vi "Spectrometer Digikröm Control Panel (No Objects).vi"(8 "error in (no error)":errorcluster) -> (0 "error out":errorcluster)   [LabVIEW 2012]
uses:
  <vilib>/Utility/error.llb/DialogType.ctl
  Digikrom DK24x/Digikrom DK24x.lvlib
panel:
  in  "exit":bool
  in  "Control":T1={"Goto Wavelength"=0.0, "Slit 1 width"=1.0000000000000004e-05, "Slit 2 width"=1.0000000000000004e-05, "Filter"=3, "Grating"=1} {"Grating" items=["Grating A"=1, "Grating B"=2, "Grating C"=3]; "Filter" items=["No filter", "Filter 1", "Filter 2", "Filter 3", "Filter 4", "Filter 5"]; "Slit 2 width" min=1.0000000000000004e-05 max=0.005000000000000002 step=1.0000000000000004e-05; "Slit 1 width" min=1.0000000000000004e-05 max=0.005000000000000002 step=1.0000000000000004e-05; "Goto Wavelength" min=0.0 max=6e-06 step=1.0000000000000008e-13 format="%.2f"}
  out "Status":T2={"Ready"=FALSE, "Wavelength"=5.000000000000003e-07, "Entrance slit"=9.999999999999999e-06, "Exit slit"=9.999999999999999e-06, " Grating (nm)"=500.0, " Filter"=0.0} {"Exit slit" format="%.2f"; "Entrance slit" format="%.2f"; "Wavelength" min=0.0 format="%.2f"}
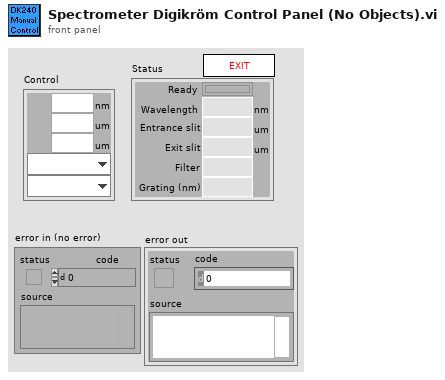
[diagram p1: front panel]
types:
  T1 = cluster{"Goto Wavelength":dbl[unit], "Slit 1 width":dbl[unit], "Slit 2 width":dbl[unit], "Filter":u32, "Grating":u16}
  T2 = cluster{"Ready":bool, "Wavelength":dbl[unit], "Entrance slit":dbl[unit], "Exit slit":dbl[unit], " Grating (nm)":dbl, " Filter":dbl}
  T3 = typedef "DialogType.ctl" = u16
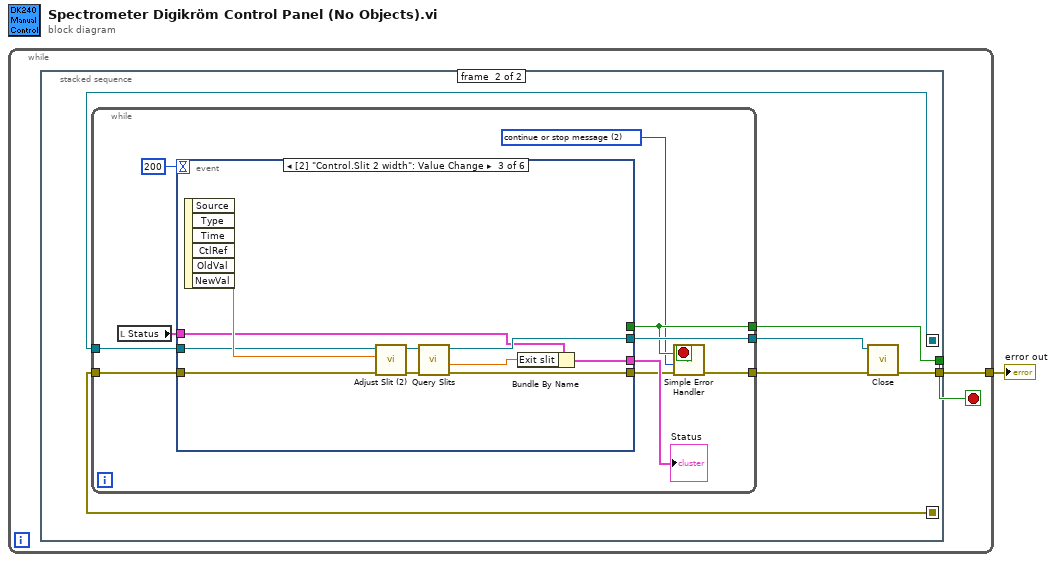
[diagram p0: block diagram]
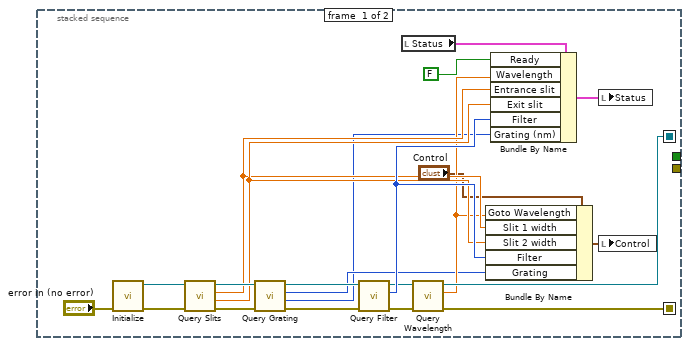
[diagram p2: hidden frame]
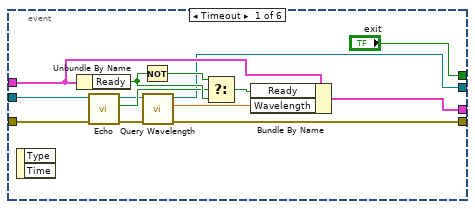
[diagram p3: hidden frame]
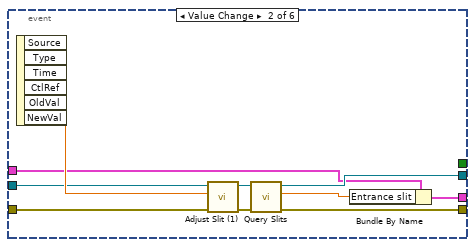
[diagram p4: hidden frame]
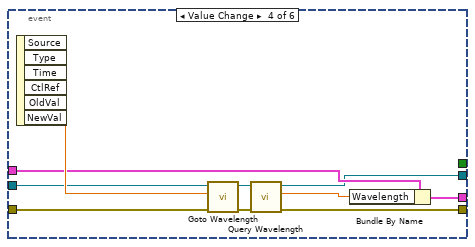
[diagram p5: hidden frame]
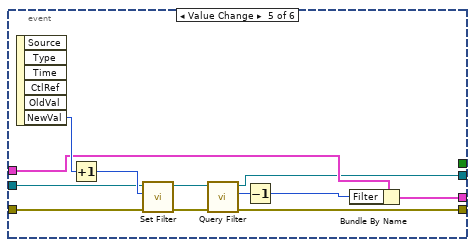
[diagram p6: hidden frame]
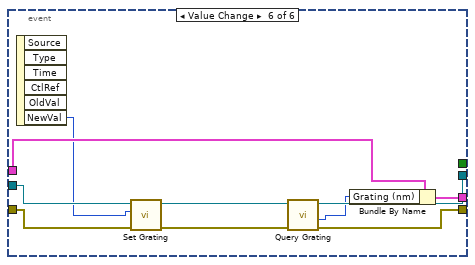
[diagram p7: hidden frame]
diagram:
  n1 = while {
    tunnel: [w2] -> w1
    stop <- w3 stop-if-true
    n2 = stacked-sequence {
      seq-local: [w18 _] -> [_ w30]
      seq-local: [w17 _] -> [_ w31]
      tunnel: [_ w29] -> w3
      tunnel: [_ w26] -> w2
      frame #0 {
        n3 = call "Initialize.vi"("error in (no error)"="error in (no error)") -> ("error out"=w22:errorcluster, "VISA resource name out"=w21:refnum<visa-resource-name>)  [unwired: 2 in, 7 out]
        n4 = call "Query Slits.vi"("error in (no error)"=w22, "VISA resource name"=w21) -> ("error out"=w19:errorcluster, "CURRENT S2 WIDTH"=w14:dbl[unit], "CURRENT S1 WIDTH"=w13:dbl[unit], "VISA resource name out"=w20:refnum<visa-resource-name>)  [unwired: 6 out]
        n5 = call "Query Grating.vi"("error in (no error)"=w19, "VISA resource name"=w20) -> ("error out"=w8:errorcluster, "BLAZE (nm)"=w6:u16, "GRATING #"=w7:u8, "VISA resource name out"=w9:refnum<visa-resource-name>)  [unwired: 6 out]
        n6 = call "Query Filter.vi"("error in (no error)"=w8, "VISA resource name"=w9) -> ("error out"=w10:errorcluster, "CURRENT FILTER"=w15:u8, "VISA resource name out"=w11:refnum<visa-resource-name>)  [unwired: 7 out]
        n7 = local read "Status"() -> (w24:T2)
        n8 = call "Query Wavelength.vi"("error in (no error)"=w10, "VISA resource name"=w11) -> ("error out"=w17:errorcluster, "CURRENT WAVELENGTH"=w12:dbl[unit], "VISA resource name out"=w18:refnum<visa-resource-name>)  [unwired: 7 out]
        n9 = Bundle By Name(cluster="Control", "Goto Wavelength"=w12, "Slit 1 width"=w13, "Slit 2 width"=w14, "Filter"=w15, "Grating"=w7) -> (w23:T1)
        n10 = Bundle By Name(cluster=w24, "Ready"=FALSE, "Wavelength"=w12, "Entrance slit"=w13, "Exit slit"=w14, "Filter"=w15, "Grating (nm)"=w6) -> (w25:T2)
        n11 = local write "Status"(w25) -> ()
        n12 = local write "Control"(w23) -> ()
      }
      frame #1 {
        n13 = while {
          tunnel: [w34] -> w29
          tunnel: w31 -> [w39]
          tunnel: [w33] -> w28
          tunnel: w30 -> [w38]
          tunnel: [w37] -> w27
          stop <- w34 stop-if-true
          w32 = T3 2 items=["no dialog", "OK message", "continue or stop message", "OK message + warnings", "continue/stop + warnings"] ("type of dialog (OK msg:1)")
          n14 = local read "Status"() -> (w35:T2)
          n15 = event shown="[2] \"Control.Slit 2 width\": Value Change" {
            selector: _ -> [_ _ _ _ _ _]
            dyn-events: _ -> [_ _ _ _ _ _]
            timeout: 200 -> [_ _ _ _ _ _]
            tunnel: ["exit" _ _ _ _ _] -> w34
            tunnel: [w55 w65 w75 w84 w96 w107] -> w41
            tunnel: w38 -> [w50 w59 w70 w81 w88 w106]
            tunnel: w39 -> [w51 w60 w71 w82 w92 w105]
            tunnel: [w45 w62 w73 w77 w86 w98] -> w36
            tunnel: [w46 w63 w74 w76 w87 w100] -> w37
            tunnel: w35 -> [w49 w58 w69 w80 w91 w104]
            event Timeout {
              n16 = event-data() -> ()  [unwired: 3 out]
              n17 = Unbundle By Name(w49) -> ("Ready"=w52:bool)
              n18 = call "Echo.vi"("error in (no error)"=w51, "VISA resource name"=w50) -> ("error out"=w44:errorcluster, "Comm OK?"=w48:bool, "VISA resource name out"=w43:refnum<visa-resource-name>)  [unwired: 7 out]
              n19 = Not(x=w52) -> (.not. x?=w53:bool)
              n20 = call "Query Wavelength.vi"("error in (no error)"=w44, "VISA resource name"=w43) -> ("error out"=w45:errorcluster, "CURRENT WAVELENGTH"=w42:dbl[unit], "VISA resource name out"=w46:refnum<visa-resource-name>)  [unwired: 7 out]
              n21 = Select(t=w53, s=w48, f=w52) -> (s? t:f=w54:bool)
              n22 = Bundle By Name(cluster=w49, "Ready"=w54, "Wavelength"=w42) -> (w55:T2)
            }
            event "Control.Slit 1 width": Value Change {
              n23 = event-data() -> ("NewVal"=w61:dbl[unit])  [unwired: 6 out]
              n24 = call "Adjust Slit (1).vi"("error in (no error)"=w60, "SLIT WIDTH"=w61, "VISA resource name"=w59) -> ("error out"=w57:errorcluster, "VISA resource name out"=w56:refnum<visa-resource-name>)  [unwired: 7 out]
              n25 = call "Query Slits.vi"("error in (no error)"=w57, "VISA resource name"=w56) -> ("error out"=w62:errorcluster, "CURRENT S1 WIDTH"=w64:dbl[unit], "VISA resource name out"=w63:refnum<visa-resource-name>)  [unwired: 7 out]
              n26 = Bundle By Name(cluster=w58, "Entrance slit"=w64) -> (w65:T2)
            }
            event "Control.Slit 2 width": Value Change {
              n27 = event-data() -> ("NewVal"=w72:dbl[unit])  [unwired: 6 out]
              n28 = call "Adjust Slit (2).vi"("error in (no error)"=w71, "SLIT WIDTH"=w72, "VISA resource name"=w70) -> ("error out"=w68:errorcluster, "VISA resource name out"=w67:refnum<visa-resource-name>)  [unwired: 7 out]
              n29 = call "Query Slits.vi"("error in (no error)"=w68, "VISA resource name"=w67) -> ("error out"=w73:errorcluster, "CURRENT S2 WIDTH"=w66:dbl[unit], "VISA resource name out"=w74:refnum<visa-resource-name>)  [unwired: 7 out]
              n30 = Bundle By Name(cluster=w69, "Exit slit"=w66) -> (w75:T2)
            }
            event "Control.Goto Wavelength": Value Change {
              n31 = event-data() -> ("NewVal"=w85:dbl[unit])  [unwired: 6 out]
              n32 = call "Goto Wavelength.vi"("error in (no error)"=w82, "WAVELENGTH"=w85, "VISA resource name"=w81) -> ("error out"=w78:errorcluster, "VISA resource name out"=w79:refnum<visa-resource-name>)  [unwired: 7 out]
              n33 = call "Query Wavelength.vi"("error in (no error)"=w78, "VISA resource name"=w79) -> ("error out"=w77:errorcluster, "CURRENT WAVELENGTH"=w83:dbl[unit], "VISA resource name out"=w76:refnum<visa-resource-name>)  [unwired: 7 out]
              n34 = Bundle By Name(cluster=w80, "Wavelength"=w83) -> (w84:T2)
            }
            event "Control.Filter": Value Change {
              n35 = event-data() -> ("NewVal"=w97:u32)  [unwired: 6 out]
              n36 = Increment(x=w97) -> (x+1=w95:u32)
              n37 = call "Set Filter.vi"("error in (no error)"=w92, "NEW FILTER"=w95, "VISA resource name"=w88) -> ("error out"=w89:errorcluster, "VISA resource name out"=w90:refnum<visa-resource-name>)  [unwired: 7 out]
              n38 = call "Query Filter.vi"("error in (no error)"=w89, "VISA resource name"=w90) -> ("error out"=w86:errorcluster, "CURRENT FILTER"=w93:u8, "VISA resource name out"=w87:refnum<visa-resource-name>)  [unwired: 7 out]
              n39 = Decrement(x=w93) -> (x-1=w94:u8)
              n40 = Bundle By Name(cluster=w91, "Filter"=w94) -> (w96:T2)
            }
            event "Control.Grating": Value Change {
              n41 = event-data() -> ("NewVal"=w103:u16)  [unwired: 6 out]
              n42 = call "Set Grating.vi"("error in (no error)"=w105, "NEW GRT?"=w103, "VISA resource name"=w106) -> ("error out"=w102:errorcluster, "VISA resource name out"=w101:refnum<visa-resource-name>)  [unwired: 7 out]
              n43 = call "Query Grating.vi"("error in (no error)"=w102, "VISA resource name"=w101) -> ("error out"=w98:errorcluster, "BLAZE (nm)"=w99:u16, "VISA resource name out"=w100:refnum<visa-resource-name>)  [unwired: 7 out]
              n44 = Bundle By Name(cluster=w104, "Grating (nm)"=w99) -> (w107:T2)
            }
          }
          "Status" <- w41
          n45 = call <vilib>:"Simple Error Handler.vi"("type of dialog (OK msg:1)"=w32, "error in (no error)"=w36) -> ("error out"=w33:errorcluster)  [unwired: 7 out]
        }
        n46 = call "Close.vi"("error in (no error)"=w28, "VISA resource name"=w27) -> ("error out"=w26:errorcluster)  [unwired: 9 out]
      }
    }
  }
  "error out" <- w1
